vi "PIDController.vi"(8 "error in (no error)":errorcluster, 11 "DAQ_QPT_Throlab in":refnum<class "DAQ_QPT_Throlab.lvclass">) -> (0 "error out":errorcluster, 3 "DAQ_QPT_Throlab out":refnum<class "DAQ_QPT_Throlab.lvclass">)   [LabVIEW 2020, in "DAQ_QPT_Throlab.lvlib" / "DAQ_QPT_Throlab.lvclass"]
uses:
  DAQ_QPT_Throlab.lvclass
  C:/Program Files/National Instruments/LabVIEW 2020/vi.lib/ActorFramework/Actor/Actor.lvclass
  DAQ_QPT_Throlab.lvclass/DAQ_QPT_Throlab.ctl
  <vilib>/ActorFramework/Actor/Actor.lvclass/Actor.ctl
  Interface/MicroscopeIO Messages/SetStagePosition Msg/SetStagePosition Msg.lvclass/SetStagePosition Msg.ctl
  <vilib>/ActorFramework/Message Enqueuer/Message Enqueuer.lvclass/Message Enqueuer.ctl
  <vilib>/ActorFramework/Message Enqueuer/Enqueue.vi
  Interface/MicroscopeIO Messages/SetStagePosition Msg/SetStagePosition Msg.lvclass
  C:/Program Files/National Instruments/LabVIEW 2020/vi.lib/ActorFramework/Message/Message.lvclass
  <vilib>/ActorFramework/Message Priority Queue/Priority Enqueue.vi
  <vilib>/ActorFramework/Actor/Actor.lvclass
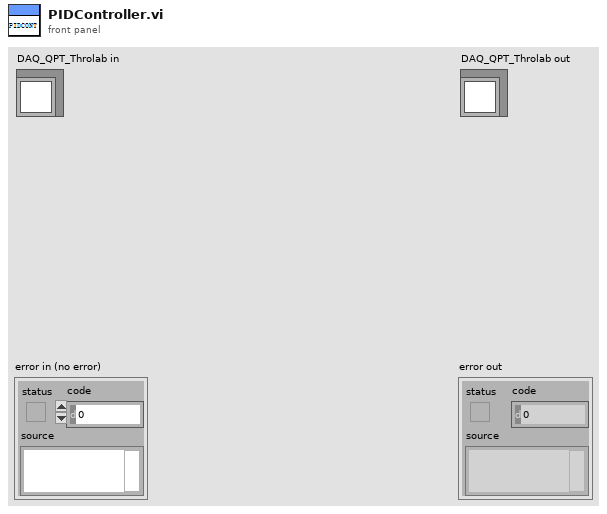
[diagram p1: front panel]
types:
  T1 = cluster{"Kp":dbl, "Ki":dbl, "Kd":dbl, "DeadZone(nm)":dbl}
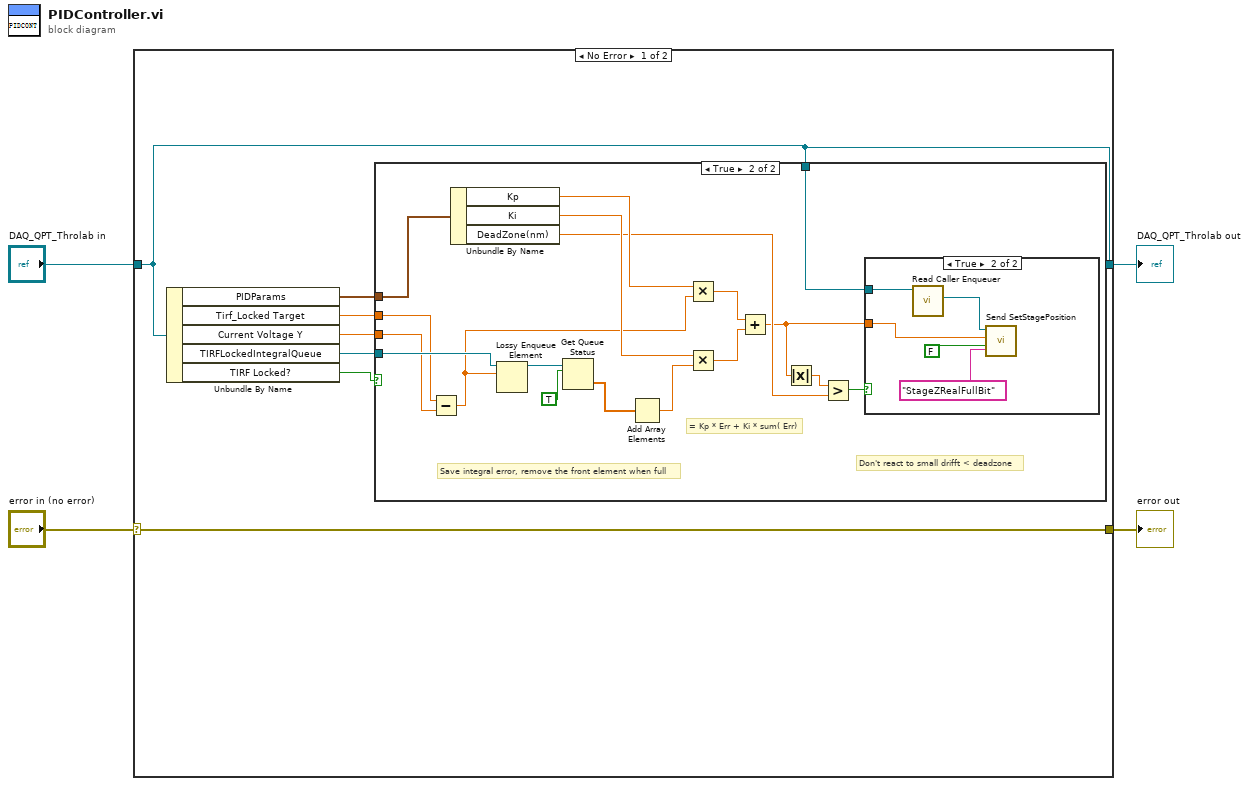
[diagram p0: block diagram]
diagram:
  n1 = case shown="No Error" "error in (no error)" {
    selector: "error in (no error)" -> [w11 w36]
    tunnel: [w11 w36] -> w3
    tunnel: [w6 w35] -> w1
    tunnel: "DAQ_QPT_Throlab in" -> [w6 w35]
    frame No Error {
      n2 = Unbundle By Name(w6) -> ("PIDParams"=w7:T1, "Tirf_Locked Target"=w9:dbl, "Current Voltage Y"=w8:dbl, "TIRFLockedIntegralQueue"=w10:refnum<queue>, "TIRF Locked?"=w5:bool)
      n3 = case shown="True" w5 {
        tunnel: w10 -> [_ w29]
        tunnel: w9 -> [_ w28]
        tunnel: w8 -> [_ w27]
        tunnel: w7 -> [_ w24]
        tunnel: w6 -> [_ w17]
        frame False {
        }
        frame True {
          # "Don't react to small drifft < deadzone"
          # "= Kp * Err + Ki * sum( Err)"
          # "Save integral error, remove the front element when full"
          n4 = Subtract(x=w28, y=w27) -> (x-y=w20:dbl)
          n5 = Unbundle By Name(w24) -> ("Kp"=w21:dbl, "Ki"=w23:dbl, "DeadZone(nm)"=w15:dbl)
          n6 = Lossy Enqueue Element(queue=w29, element=w20) -> (queue out=w26:refnum<queue>)  [unwired: 1 in, 3 out]
          n7 = Get Queue Status(queue=w26, return elements? (F)=TRUE) -> (elements=w25:dbl[])  [unwired: 1 in, 7 out]
          n8 = Add Array Elements(numeric array=w25) -> (sum=w22:dbl)
          n9 = Multiply(x=w21, y=w20) -> (x*y=w19:dbl)
          n10 = Multiply(x=w23, y=w22) -> (x*y=w18:dbl)
          n11 = Add(x=w19, y=w18) -> (x+y=w13:dbl)
          n12 = Absolute Value(x=w13) -> (abs(x)=w12:dbl)
          n13 = Greater?(x=w12, y=w15) -> (0:w14:bool)
          n14 = case shown="True" w14 {
            tunnel: w17 -> [_ w34]
            tunnel: w13 -> [_ w30]
            frame False {
            }
            frame True {
              n15 = call <vilib>:"Read Caller Enqueuer.vi"("Actor"=w34) -> ("Caller Enqueuer"=w33:refnum<class "Message Enqueuer.lvclass">)  [unwired: 10 in]
              n16 = call "Send SetStagePosition.vi"("Label"="StageZRealFullBit", "AbsPosition?"=FALSE, "Value"=w30, "Message Enqueuer"=w33) -> ()  [unwired: 6 in, 2 out]
            }
          }
        }
      }
    }
    frame Error {
    }
  }
  "error out" <- w3
  "DAQ_QPT_Throlab out" <- w1
